vi "Fetch Waveforms.vi"(8 "error in (no error)":errorcluster, 11 "Thermometer DAQmx in":refnum<class "Thermometer DAQmx.lvclass">) -> (0 "error out":errorcluster, 3 "Thermometer DAQmx out":refnum<class "Thermometer DAQmx.lvclass">)   [LabVIEW 2023, in "Thermometer.lvlib" / "Thermometer DAQmx.lvlib" / "Thermometer DAQmx.lvclass"]
uses:
  Thermometer DAQmx.lvclass
  Interfaces/IConfigure IAI/IConfigure IAI.lvclass
  Thermometer Base/Thermometer Base.lvclass/Thermometer Base.ctl
  Thermometer DAQmx.lvclass/Thermometer DAQmx.ctl
  Thermometer Base/Thermometer Base.lvclass
  D:/git/HAL/Thermometer/Thermometer Base/Thermometer Base.lvclass
  D:/git/HAL/Instrument/Instrument.lvclass
  D:/git/HAL/Interfaces/IThermometer/IThermometer.lvclass
  D:/git/HAL/Thermometer/Thermometer DAQmx/Thermometer DAQmx/Thermometer DAQmx.lvclass
  D:/git/HAL/Interfaces/IAI/IAI.lvclass
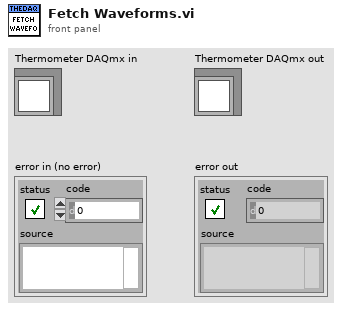
[diagram p1: front panel]
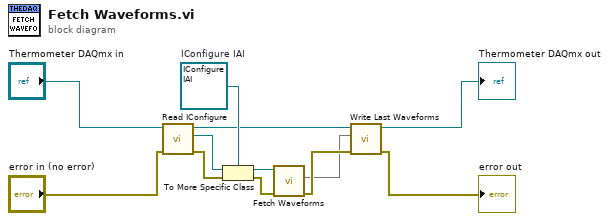
[diagram p0: block diagram]
diagram:
  w7 = refnum<class "IConfigure IAI.lvclass"> refnum  # IConfigure IAI
  n1 = call "Read IConfigure.vi"("error in (no error)"="error in (no error)", "Thermometer Base in"="Thermometer DAQmx in") -> ("error out"=w10:errorcluster, "IConfigure"=w12:refnum<class "IConfigure.lvclass">, "Thermometer Base out"=w6:refnum<class "Thermometer DAQmx.lvclass">)  [unwired: 7 in]
  n2 = To More Specific Class(target class=w7, reference=w12, error in=w10) -> (specific class reference=w8:refnum<class "IConfigure IAI.lvclass">, error out=w9:errorcluster)
  n3 = call-dynamic "Fetch Waveforms.vi"("error in (no error)"=w9, "IConfigure IAI in"=w8) -> ("error out"=w11:errorcluster, "Last Waveforms"=w5:map{u8, waveform(dbl)})  [unwired: 7 in, 1 out]
  n4 = call "Write Last Waveforms.vi"("error in (no error)"=w11, "Last Waveforms"=w5, "Thermometer DAQmx in"=w6) -> ("error out"=→"error out":errorcluster, "Thermometer DAQmx out"=→"Thermometer DAQmx out":refnum<class "Thermometer DAQmx.lvclass">)  [unwired: 7 in]
